vi "Histogram.vi"() -> ()   [LabVIEW 2015]
uses:
  <vilib>/Utility/file.llb/Read Delimited Spreadsheet (DBL).vi
  <vilib>/Analysis/NI_AALBase.lvlib
panel:
  out "Histogram":T1(graph)
  out "Veriler":dbl[][](array[numeric])
  in  "Okunacak Veri Adresi":path
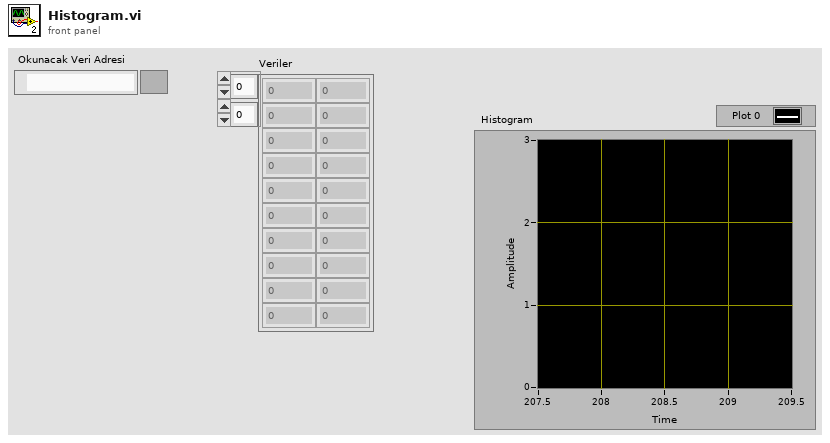
[diagram p1: front panel]
types:
  T1 = cluster{"X Values":dbl[], "Histogram: h(x)":i32[]}
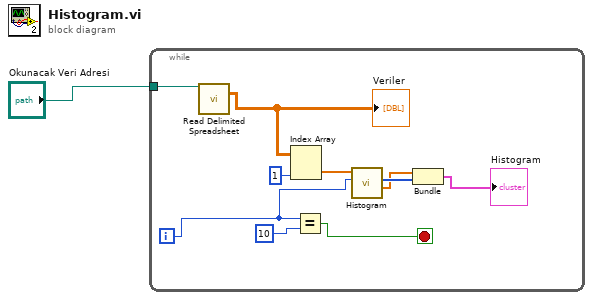
[diagram p0: block diagram]
diagram:
  n1 = while {
    tunnel: "Okunacak Veri Adresi" -> [w11]
    i -> [w2]
    stop <- w8 stop-if-true
    n2 = call-poly <vilib>:"Read Delimited Spreadsheet.vi"("file path (dialog if empty)"=w11) -> ("all rows"=w10:dbl[][])  [unwired: 9 in, 5 out]
    "Veriler" <- w10
    n3 = Index Array(array=w10, index (col)=1 ("disabled index (col)")) -> (element=w6:dbl[])  [unwired: 1 in]
    n4 = Equal?(x=w2, y=10) -> (x = y?=w8:bool)
    n5 = call <vilib>:"Histogram.vi"("intervals"=w2, "X"=w6) -> ("X Values"=w4:dbl[], "Histogram: h(x)"=w5:i32[])  [unwired: 6 in, 2 out]
    n6 = Bundle("X Values"=w4, "Histogram: h(x)"=w5) -> (→"Histogram":T1)  [unwired: 1 in]
  }
